vi "Read Numeric Refnum.vi"(8 "error in (no error)":errorcluster, 11 "Numeric Field in":refnum<class "Numeric Field.lvclass">) -> (0 "error out":errorcluster, 2 "Num Refnum":refnum<vi>, 3 "Numeric Field out":refnum<class "Numeric Field.lvclass">)   [LabVIEW 2020, in "Numeric Field.lvclass"]
uses:
  Numeric Field.lvclass
  C:/Users/User/Desktop/Raman Program/Database OOP/source/Field/Field.lvclass
  Field.lvclass/Field.ctl
  Field.lvclass
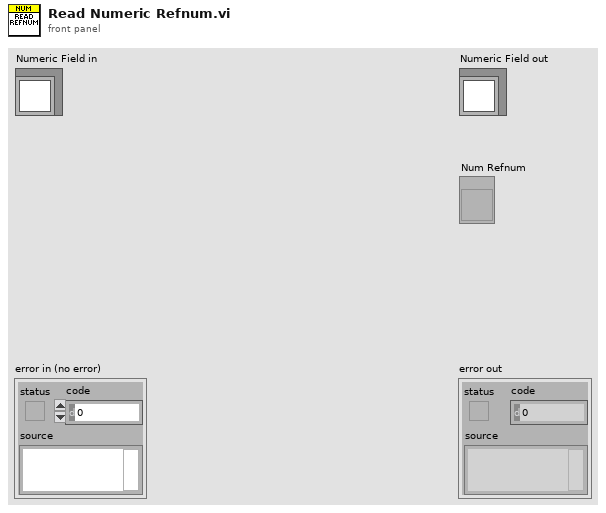
[diagram p1: front panel]
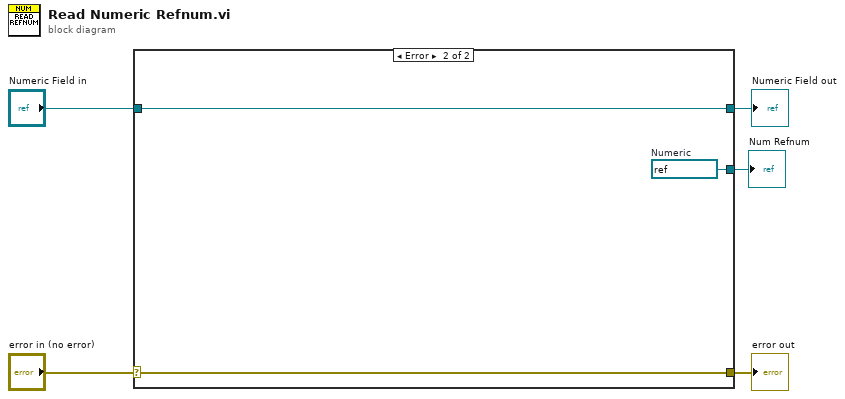
[diagram p0: block diagram]
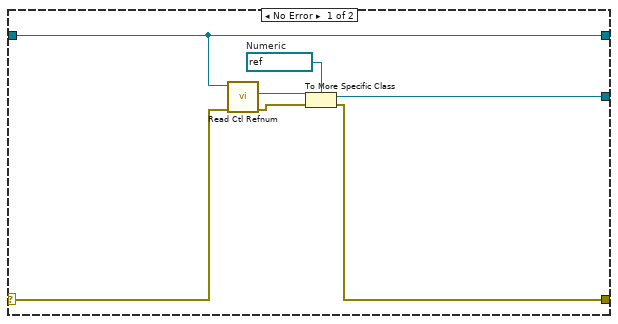
[diagram p2: hidden frame]
diagram:
  n1 = case shown="Error" "error in (no error)" {
    selector: "error in (no error)" -> [w9 w15]
    tunnel: [w7 w15] -> w4
    tunnel: [w12 w14] -> w2
    tunnel: "Numeric Field in" -> [w12 w14]
    tunnel: [w6 w13] -> w1
    frame No Error {
      w10 = refnum<vi> refnum  # Numeric
      n2 = call "Read Ctl Refnum.vi"("error in (no error)"=w9, "Field in"=w12) -> ("error out"=w8:errorcluster, "Ctl Refnum"=w11:refnum<vi>)  [unwired: 7 in, 1 out]
      n3 = To More Specific Class(target class=w10, reference=w11, error in=w8) -> (specific class reference=w6:refnum<vi>, error out=w7:errorcluster)
    }
    frame Error {
      w13 = refnum<vi> refnum  # Numeric
    }
  }
  "error out" <- w4
  "Numeric Field out" <- w2
  "Num Refnum" <- w1
